vi "Pressure2PSI.vi"(9 "Unit":string, 10 "Numeric":dbl) -> (2 "PSI":dbl)   [LabVIEW 2012]
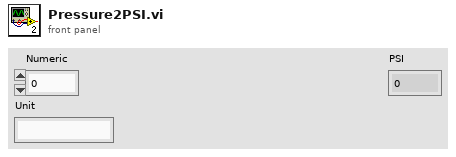
[diagram p1: front panel]
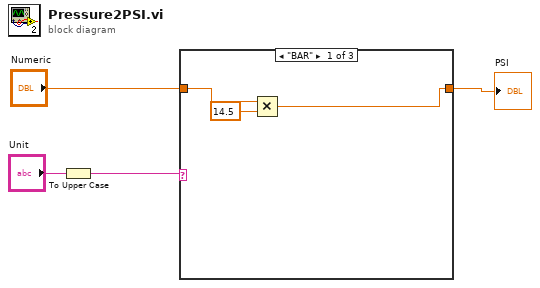
[diagram p0: block diagram]
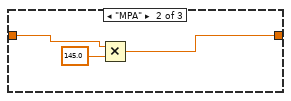
[diagram p2: hidden frame]
diagram:
  n1 = To Upper Case(1:"Unit") -> (0:w1:string)
  n2 = case shown="\"BAR\"" w1 {
    tunnel: "Numeric" -> [w7 w10 w11]
    tunnel: [w5 w8 w11] -> w2
    frame "BAR" {
      n3 = Multiply(x=w7, y=14.5) -> (x*y=w5:dbl)
    }
    frame "MPA" {
      n4 = Multiply(x=w10, y=145.0) -> (x*y=w8:dbl)
    }
    frame "PSI", Default {
    }
  }
  "PSI" <- w2
